vi "Timed Structure Offset.vi"(11 "delayInSeconds":dbl=3.0) -> (3 "TimeStamp":timestamp)   [LabVIEW 2020]
uses:
  <vilib>/Platform/TimedLoop/XDataNode/timing_clust.ctl
  <vilib>/Platform/TimedLoop/XDataNode/nitl_modes.ctl
  <vilib>/Platform/TimedLoop/XDataNode/wakeup.ctl
  <vilib>/Platform/TimedLoop/TimeConversion.llb/rt-timestamp-to-milliseconds.vi
  <vilib>/platform/TimedLoop/XDataNode/XDataNode.xnode
  <vilib>/Platform/TimedLoop/XDataNode/XDNodeRunTimeDep.lvlib
panel:
  out "StartTime":timestamp
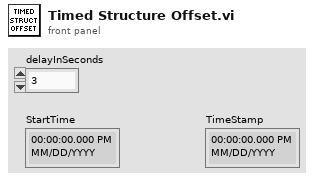
[diagram p1: front panel]
types:
  T1 = typedef "XDNodeRunTimeDep.lvlib/timing_clust.ctl" = cluster{"Expected End [f-1]":u64, "Actual End [f-1]":u64, "Finished Late? [f-1]":bool, "Expected End [i-1]":u64, "Actual End [i-1]":u64, "Finished Late? [i-1]":bool, "Expected Start [i]":u64, "Actual Start [i]":u64, "Expected Start [f]":u64, "Actual Start [f]":u64, "Source Name":string, "Structure Name":string, "Period":i64, "Deadline":i64, "Offset":i64, "Start":i64, "Priority":i32, "Timeout":i32, "Mode":T2, "Wakeup Reason":T3, "Error":errorcluster, "Source Type":string, "Secondary Source Type":string, "Global End Time":u64, "Global Start Time":u64, "Frame Duration":u64, "Iteration Duration":u64, "Assigned CPU":i32, "I/O Scan Engine Mode":u32}
  T2 = typedef "XDNodeRunTimeDep.lvlib/nitl_modes.ctl" = enum32{"No Change", "Process missed periods, maintain original phase", "Discard missed periods, maintain original phase", "Process missed periods, ignore original phase", "Discard missed periods, ignore original phase"}
  T3 = typedef "XDNodeRunTimeDep.lvlib/wakeup.ctl" = enum32{"Normal", "Aborted", "Asynchronous wakeup", "Timing source error", "Timed loop error", "Timeout"}
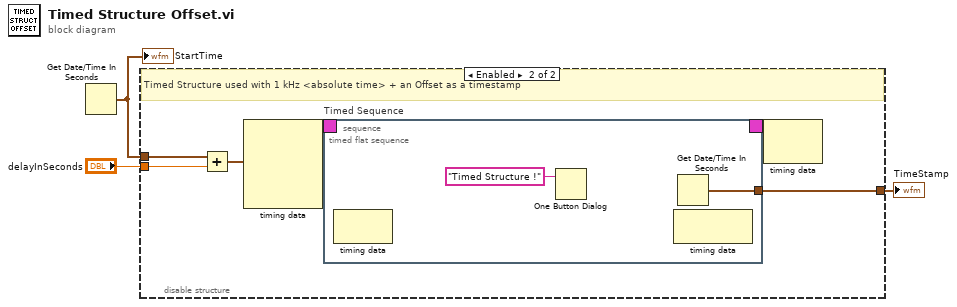
[diagram p0: block diagram]
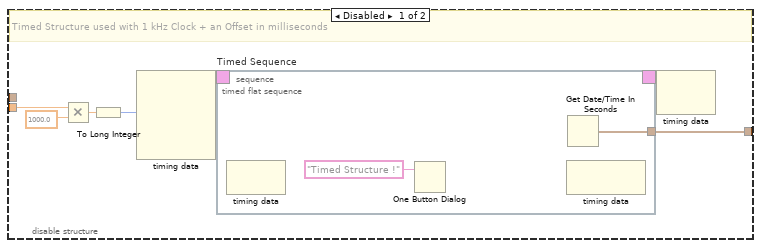
[diagram p2: hidden frame]
diagram:
  n1 = Get Date/Time In Seconds() -> (seconds since 1Jan1904=w1:timestamp)
  "StartTime" <- w1
  n2 = disable-structure shown="Enabled" {
    disable-tunnel: "delayInSeconds" -> [w6 w23]
    disable-tunnel: [w4 w21] -> w2
    disable-tunnel: w1 -> [_ w20]
    frame Disabled {
      # "Timed Structure used with 1 kHz Clock + an Offset in milliseconds"
      n3 = Multiply(x=w6, y=1000.0) -> (x*y=w8:dbl)
      n4 = To Long Integer(number=w8) -> (32bit integer=w5:i32)
      n5 = node-c288(w5) -> (w10:T1)  [unwired: 3 in]
      n6 = timed-sequence "Timed Sequence" {
        timing: w10 -> [_]
        timing-out: [_] -> w9
        tunnel: [w11] -> w4
        n7 = timed-flat-sequence {
          tunnel: [w12] -> w11
          n8 = node-c288() -> ()  [unwired: 1 in, 1 out]
          n9 = One Button Dialog(message="Timed Structure !") -> ()  [unwired: 1 in, 1 out]
          n10 = node-c288() -> ()  [unwired: 1 in, 1 out]
          n11 = Get Date/Time In Seconds() -> (seconds since 1Jan1904=w12:timestamp)
        }
      }
      n12 = node-c288(w9) -> ()  [unwired: 1 out]
    }
    frame Enabled {
      # "Timed Structure used with 1 kHz <absolute time> + an Offset as a timestamp"
      n13 = Add(x=w20, y=w23) -> (x+y=w22:timestamp)
      n14 = node-c288(w22) -> (w25:T1)  [unwired: 3 in]
      n15 = timed-sequence "Timed Sequence" {
        timing: w25 -> [_]
        timing-out: [_] -> w24
        tunnel: [w26] -> w21
        n16 = timed-flat-sequence {
          tunnel: [w27] -> w26
          n17 = node-c288() -> ()  [unwired: 1 in, 1 out]
          n18 = One Button Dialog(message="Timed Structure !") -> ()  [unwired: 1 in, 1 out]
          n19 = node-c288() -> ()  [unwired: 1 in, 1 out]
          n20 = Get Date/Time In Seconds() -> (seconds since 1Jan1904=w27:timestamp)
        }
      }
      n21 = node-c288(w24) -> ()  [unwired: 1 out]
    }
  }
  "TimeStamp" <- w2
